vi "Generate DC Offset Sequence.vi"(8 "error in (no error)":errorcluster, 11 "Device in":refnum<class "Device.lvclass">) -> (0 "error out":errorcluster, 3 "Device out":refnum<class "Device.lvclass">)   [LabVIEW 2020, in "Device.lvclass"]
uses:
  Device.lvclass
  Instruments/Power Supply/Power Supply.lvclass
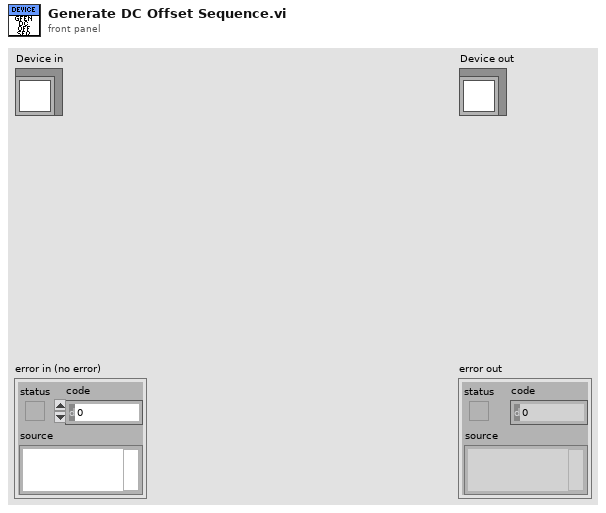
[diagram p1: front panel]
types:
  T1 = typedef "Device.lvclass/DC Offset Cluster.ctl" = cluster{"Enable":bool, "Use Array":bool, "Array":dbl[], "To From Cluster":cluster{"From":dbl, "To":dbl, "Step":dbl}, "Current Value":dbl, "DC Offset":refnum<class "Power Supply.lvclass">}
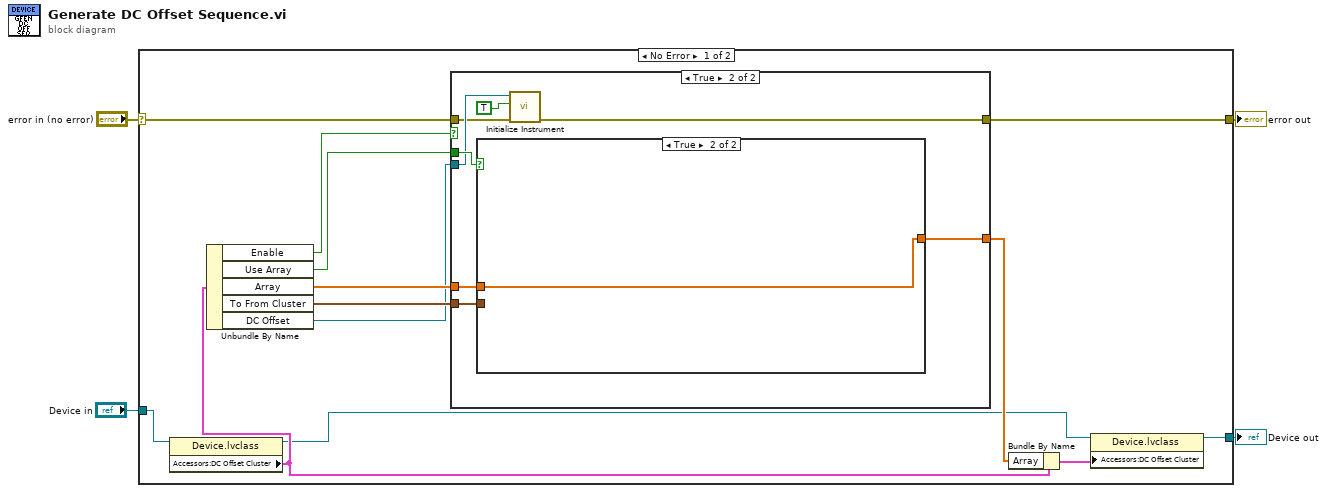
[diagram p0: block diagram]
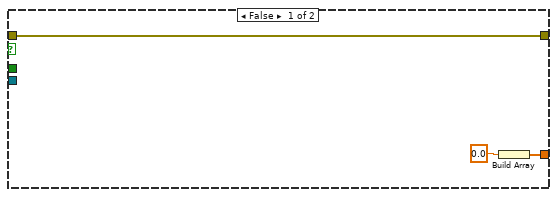
[diagram p2: hidden frame]
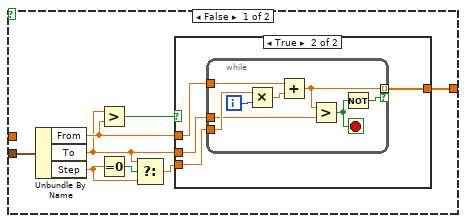
[diagram p3: hidden frame]
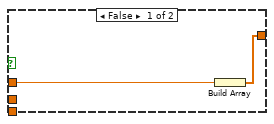
[diagram p4: hidden frame]
diagram:
  n1 = case shown="No Error" "error in (no error)" {
    selector: "error in (no error)" -> [w14 w53]
    tunnel: [w13 w53] -> w3
    tunnel: [w5 w52] -> w1
    tunnel: "Device in" -> [w9 w52]
    frame No Error {
      n2 = property class="Device.lvclass"(reference=w9) -> (reference out=w7:refnum<class "Device.lvclass">, "Accessors:DC Offset Cluster"=w8:T1)  [unwired: 1 in, 1 out]
      n3 = Unbundle By Name(w8) -> ("Enable"=w10:bool, "Use Array"=w17:bool, "Array"=w16:dbl[], "To From Cluster"=w15:cluster{"From":dbl, "To":dbl, "Step":dbl}, "DC Offset"=w11:refnum<class "Power Supply.lvclass">)
      n4 = case shown="True" w10 {
        tunnel: w17 -> [_ w28]
        tunnel: w16 -> [_ w27]
        tunnel: w15 -> [_ w26]
        tunnel: w11 -> [_ w24]
        tunnel: [w19 w25] -> w12
        tunnel: w14 -> [w18 w23]
        tunnel: [w18 w21] -> w13
        frame False {
          n5 = Build Array(0.0) -> (w19:dbl[])
        }
        frame True {
          n6 = case shown="True" w28 {
            tunnel: [w29 w51] -> w25
            tunnel: w27 -> [_ w51]
            tunnel: w26 -> [w30 _]
            frame False {
              n7 = Unbundle By Name(w30) -> ("From"=w35:dbl, "To"=w34:dbl, "Step"=w32:dbl)
              n8 = Greater?(x=w34, y=w35) -> (0:w36:bool)
              n9 = Equal To 0?(x=w32) -> (x = 0?=w31:bool)
              n10 = Select(t=w34, s=w31, f=w32) -> (s? t:f=w33:dbl)
              n11 = case shown="True" w36 {
                tunnel: [w37 w42] -> w29
                tunnel: w33 -> [_ w41]
                tunnel: w34 -> [_ w40]
                tunnel: w35 -> [w38 w39]
                frame False {
                  n12 = Build Array(w38) -> (w37:dbl[])
                }
                frame True {
                  n13 = while {
                    tunnel: w40 -> [w45]
                    tunnel: w41 -> [w48]
                    tunnel: [w46] -> w42 mode=indexing if=w44
                    tunnel: w39 -> [w50]
                    i -> [w49]
                    stop <- w43 stop-if-true
                    n14 = Multiply(x=w48, y=w49) -> (x*y=w47:dbl)
                    n15 = Add(x=w50, y=w47) -> (x+y=w46:dbl)
                    n16 = Greater?(x=w46, y=w45) -> (0:w43:bool)
                    n17 = Not(x=w43) -> (.not. x?=w44:bool)
                  }
                }
              }
            }
            frame True {
            }
          }
          n18 = call-dynamic "Initialize Instrument.vi"("error in (no error)"=w23, "Reset"=TRUE, "Power Supply in"=w24) -> ("error out"=w21:errorcluster)  [unwired: 7 in, 1 out]
        }
      }
      n19 = Bundle By Name(cluster=w8, "Array"=w12) -> (w6:T1)
      n20 = property class="Device.lvclass"(reference=w7, "Accessors:DC Offset Cluster"=w6) -> (reference out=w5:refnum<class "Device.lvclass">)  [unwired: 1 in, 1 out]
    }
    frame Error {
    }
  }
  "error out" <- w3
  "Device out" <- w1
